vi "process_DAQ.vi"() -> ()   [LabVIEW 2011, in "Fiberscope_library.lvlib"]
uses:
  Fiberscope_library.lvlib
  typedefs/control_process_state_cluster.ctl
  typedefs/control_process_state_enum.ctl
  typedefs/fpga_main_spiral_fpga_ref.ctl
  typedefs/element_streams_cluster.ctl
  typedefs/feedback_to_watchdog.ctl
  typedefs/feedback_from_process_enum.ctl
  fpga/typedefs/pixel_to_host_enum.ctl
  typedefs/run_mode_enum.ctl
  typedefs/main_state_cluster.ctl
  typedefs/main_state_enum.ctl
  typedefs/all_scan_parameters_cluster.ctl
  typedefs/fiber_parameters_cluster.ctl
  fpga/typedefs/ramp_type_enum.ctl
  typedefs/spiral_parameters_cluster.ctl
  typedefs/run_parameters_cluster.ctl
  typedefs/acquisition_parameters_cluster.ctl
  typedefs/image_size_I32.ctl
  typedefs/smooth_coeffs_cluster.ctl
  typedefs/storage_parameters_cluster.ctl
  typedefs/mapping_corrections_cluster.ctl
  typedefs/pockels_corrections_cluster.ctl
  <vilib>/Utility/error.llb/Error Cluster From Error Code.vi
  <vilib>/rvi/errors/niLvFpgaAdjustHostInterfaceError.vi
  <vilib>/FPGAPlugInAG/PXI-7813R/niLvFpga_Reset_PXI-7813R.vi
  <vilib>/rvi/interface/nirviReadWriteControl/nirviReadWriteControl.xnode
  FPGA Bitfiles/FiberscopeRK1107_FPGATarget_fpgamainspiral_0DF2A7CB.lvbitx
  <vilib>/rvi/interface/nirviMethod/nirviMethod.xnode
  <vilib>/FPGAPlugInAG/PXI-7813R/niLvFpga_ConfigureFifo_PXI-7813R.vi
  <vilib>/rvi/errors/niLvFpgaMergeErrorWithErrorCode.vi
  NiFpgaLv.dll
panel:
  out "Forth or back?":bool
  out "Frame no":u32
  out "Elements remaining in FIFO":cluster{"Ch0":u32, "Ch1":u32}
  out "Pixels per frame":u32=1 min=1 max=90000 step=1
  out "error out":errorcluster
  in  "error in":errorcluster
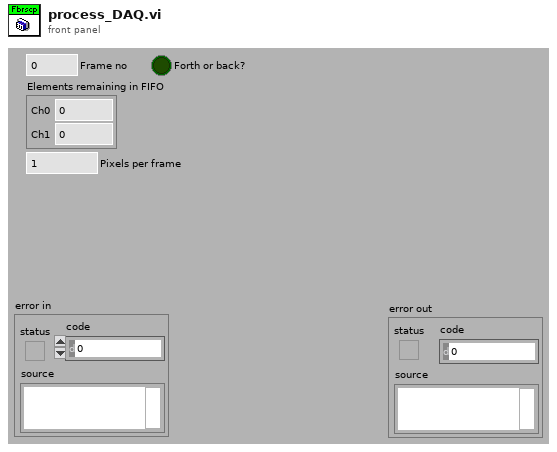
[diagram p1: front panel]
types:
  T1 = typedef "Fiberscope_library.lvlib/feedback_to_watchdog.ctl" = cluster{"Feedback_from_process_enum":T2, "Process_name":string}
  T2 = typedef "Fiberscope_library.lvlib/feedback_from_process_enum.ctl" = enum16{"Has_initialised", "Changed_parameters", "Has_started", "Has_stopped", "Has_quitted", "Is_running", "Has_finished", "Custom"}
  T3 = typedef "Fiberscope_library.lvlib/fpga_main_spiral_fpga_ref.ctl" = refnum<k20>
  T4 = typedef "Fiberscope_library.lvlib/control_process_state_cluster.ctl" = cluster{"Control_process_state_enum":T5, "variant":variant}
  T5 = typedef "Fiberscope_library.lvlib/control_process_state_enum.ctl" = enum16{"Init", "Quit", "Start", "Stop", "Change_parameters", "Running", "Finish", "Custom"}
  T6 = typedef "Fiberscope_library.lvlib/element_streams_cluster.ctl" = cluster{"Streams_array":dbl[][], "#channels":i32, "Last element?":bool, "Forth (1) or back (0)?":bool}
  T7 = typedef "pixel_to_host_enum.ctl" = enum16{"four-channel mode", "two-channel mode"}
  T8 = typedef "Fiberscope_library.lvlib/main_state_cluster.ctl" = cluster{"Main_state_enum":T9, "State_data_variant":variant}
  T9 = typedef "Fiberscope_library.lvlib/main_state_enum.ctl" = enum16{"Init", "Error", "Quit", "Run", "Stop", "Change_parameters", "Timeout", "Shutter", "Save", "Wait_for_finished", "Change_storage", "Change_pixelmap", "Change_averages", "Run_finished", "Change_runmode", "PMT"}
  T10 = typedef "Fiberscope_library.lvlib/run_mode_enum.ctl" = enum16{"Continuous", "Single frame", "No. of frames"}
  T11 = typedef "Fiberscope_library.lvlib/all_scan_parameters_cluster.ctl" = cluster{"Fiber parameters":T12, "Spiral parameters":T14, "Run parameters":T15, "Acquisition parameters":T16, "Fiber parameters pixel_mapper":T12, "Smooth_coeffs_cluster":T18, "Storage parameters":T19, "Mapping corrections":T20, "Pockels corrections":T21}
  T12 = typedef "Fiberscope_library.lvlib/fiber_parameters_cluster.ctl" = cluster{"Frequency":dbl, "Amplitude X":dbl, "Amplitude Y":dbl, "Initial Amplitude X":dbl, "Initial Amplitude Y":dbl, "Phase":dbl, "Ramp type":T13}
  T13 = typedef "ramp_type_enum.ctl" = enum8{"Linear", "Sine"}
  T14 = typedef "Fiberscope_library.lvlib/spiral_parameters_cluster.ctl" = cluster{"Imaging periods":dbl, "Settling periods":dbl, "Resting periods":dbl}
  T15 = typedef "Fiberscope_library.lvlib/run_parameters_cluster.ctl" = cluster{"Run mode":T10, "Averages per frame":u8, "No. of frames":u32}
  T16 = typedef "Fiberscope_library.lvlib/acquisition_parameters_cluster.ctl" = cluster{"Cycles per pixel":u32, "Image size":T17, "Bidirectional acquisition":bool}
  T17 = typedef "Fiberscope_library.lvlib/image_size_I32.ctl" = i32
  T18 = typedef "Fiberscope_library.lvlib/smooth_coeffs_cluster.ctl" = cluster{"Coeff 1":dbl, "Coeff 2":dbl}
  T19 = typedef "Fiberscope_library.lvlib/storage_parameters_cluster.ctl" = cluster{"Autosave":bool, "Path":path}
  T20 = typedef "Fiberscope_library.lvlib/mapping_corrections_cluster.ctl" = cluster{"Phase increase":dbl, "Amplitude correction":dbl}
  T21 = typedef "Fiberscope_library.lvlib/pockels_corrections_cluster.ctl" = cluster{"Delay pixels":i32}
  T22 = cluster{"Elements Remaining":u32, "Elements Remaining":u32}
  T23 = typedef "Fiberscope_library.lvlib/FPGA_acquisition_parameters.ctl" = cluster{"Cycles per pixel":u32, "Bitshift":i8, "Bidirectional acquisition":bool}
  T24 = typedef "scan_parameters_cluster.ctl" = cluster{"No. of waveforms":u16, "Continuous scanning":bool}
  T25 = typedef "cycle_parameters_XY_cluster.ctl" = cluster{"Cycle parameters X":T26, "Cycle parameters Y":T26}
  T26 = typedef "cycle_parameters_cluster.ctl" = cluster{"Imaging cycles":i32, "Settling cycles":i32, "Resting cycles":i32, "Phase advance per cycle":fxp<+,32,0>, "Initial Phase":fxp<+,32,1>}
  T27 = typedef "ramp_parameters_XY_cluster.ctl" = cluster{"Ramp parameters X":T28, "Ramp parameters Y":T28}
  T28 = typedef "ramp_parameters_cluster.ctl" = cluster{"Ramp type":T13, "Linear ramp parameters":T29, "Sine ramp parameters":T30}
  T29 = typedef "linear_ramp_parameters_cluster.ctl" = cluster{"Imaging multiplier advance per cycle":fxp<+/-,32,0>, "Settling multiplier advance per cycle":fxp<+/-,32,0>, "Imaging initial multiplier":fxp<+/-,43,12>}
  T30 = typedef "sine_ramp_parameters_cluster.ctl" = cluster{"Imaging phase advance per cycle":fxp<+,32,0>, "Settling phase advance per cycle":fxp<+,32,0>, "Scaler":fxp<+,43,12>, "Imaging initial phase":fxp<+,32,1>}
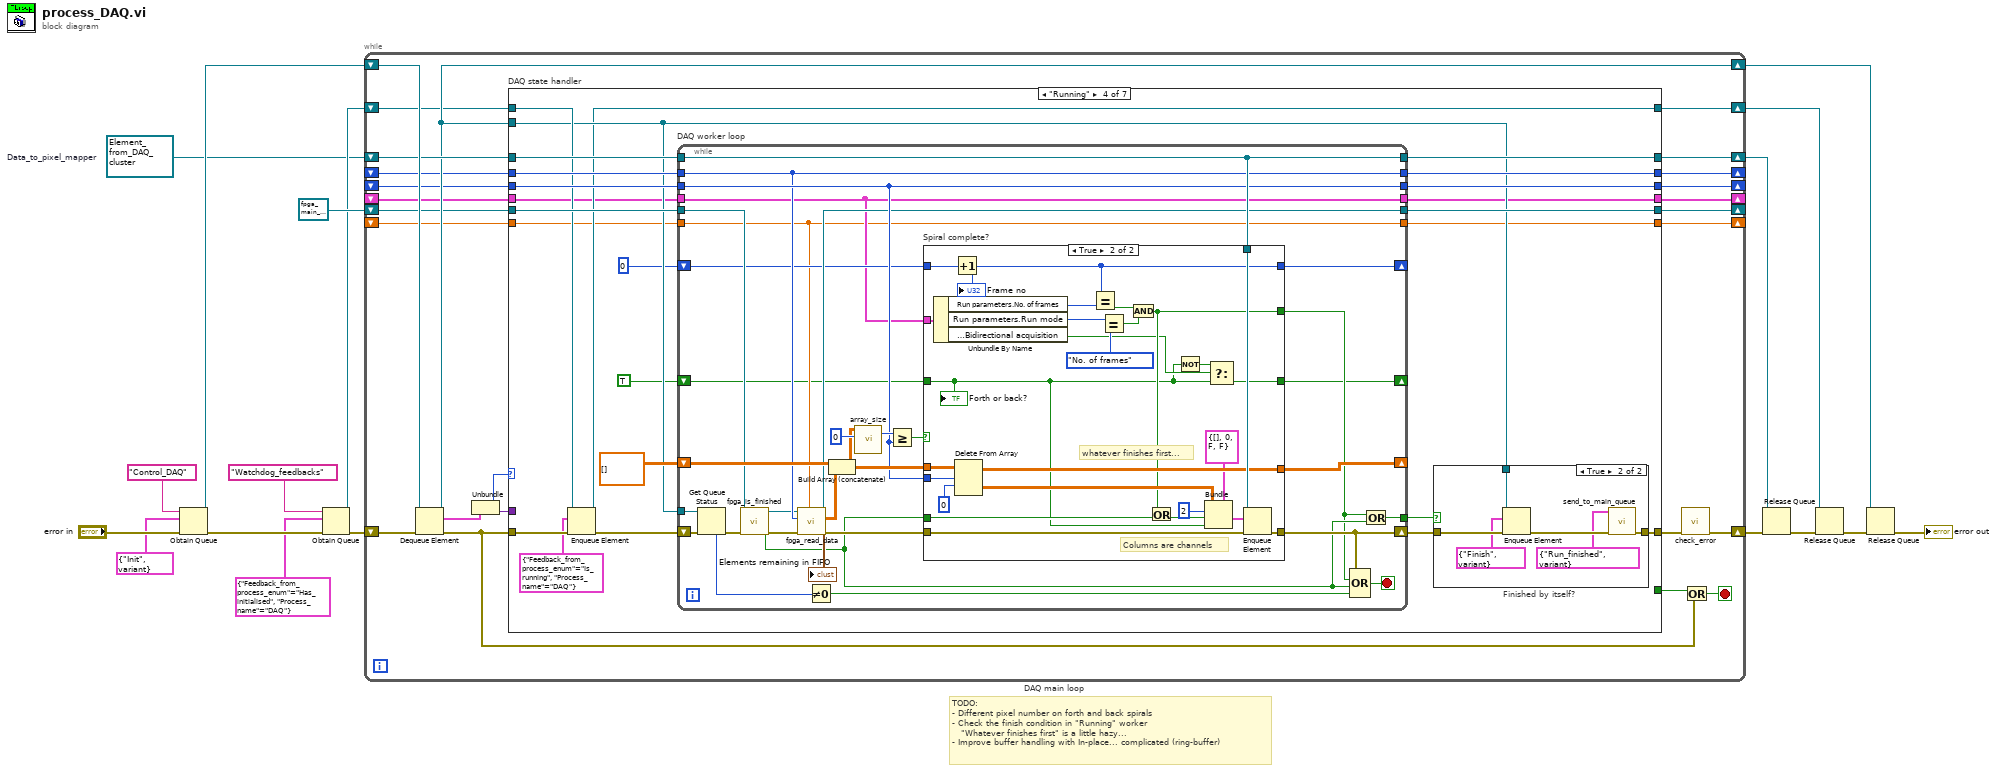
[diagram p0: block diagram]
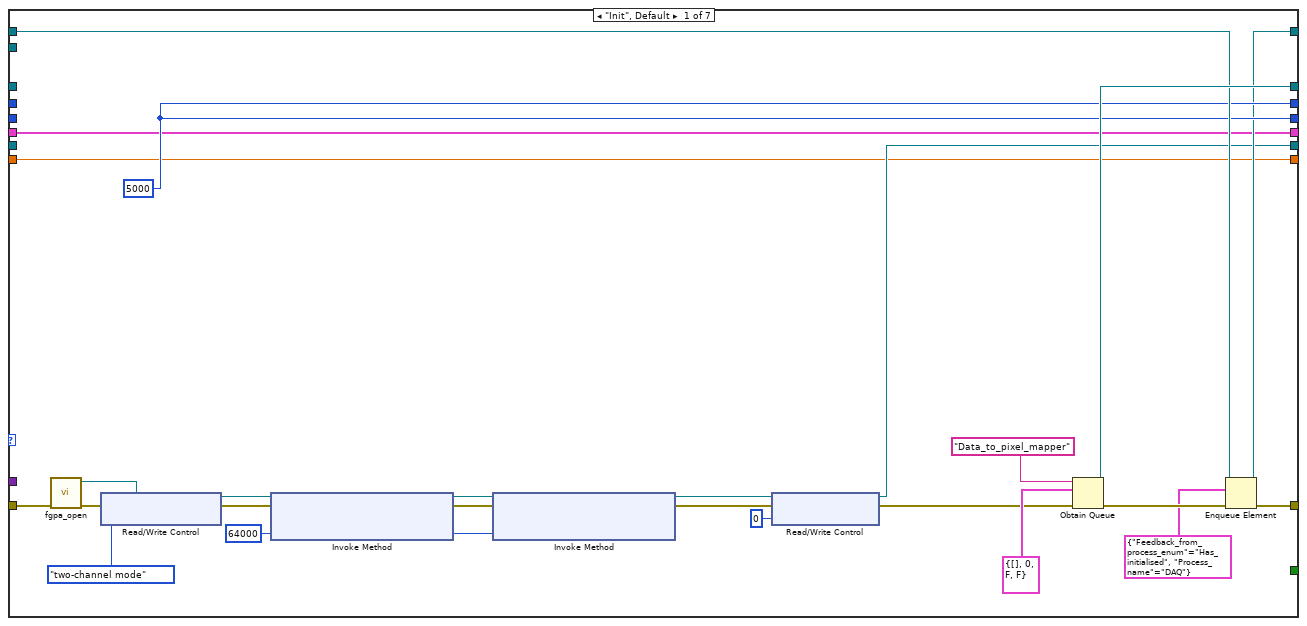
[diagram p2: hidden frame]
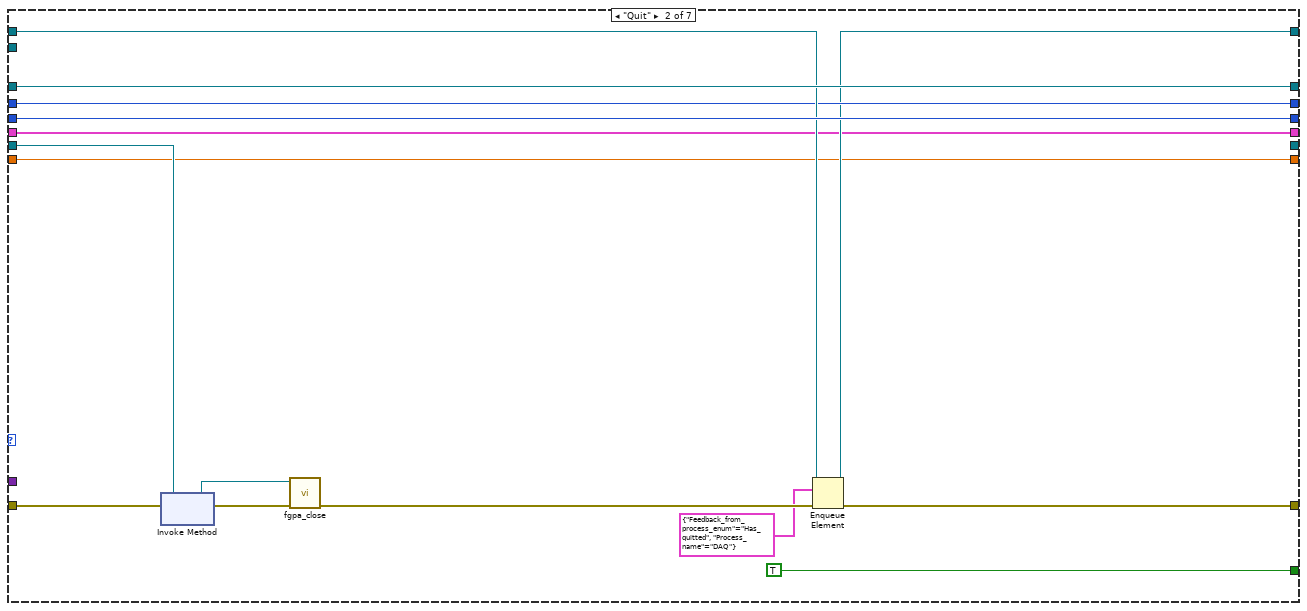
[diagram p3: hidden frame]
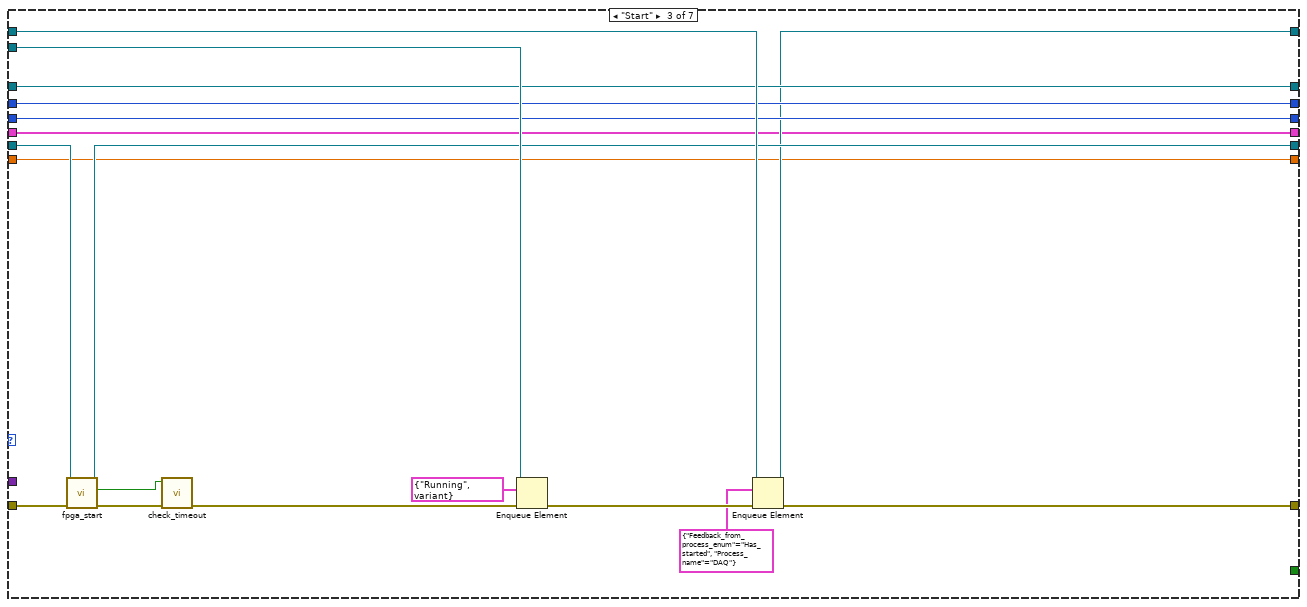
[diagram p4: hidden frame]
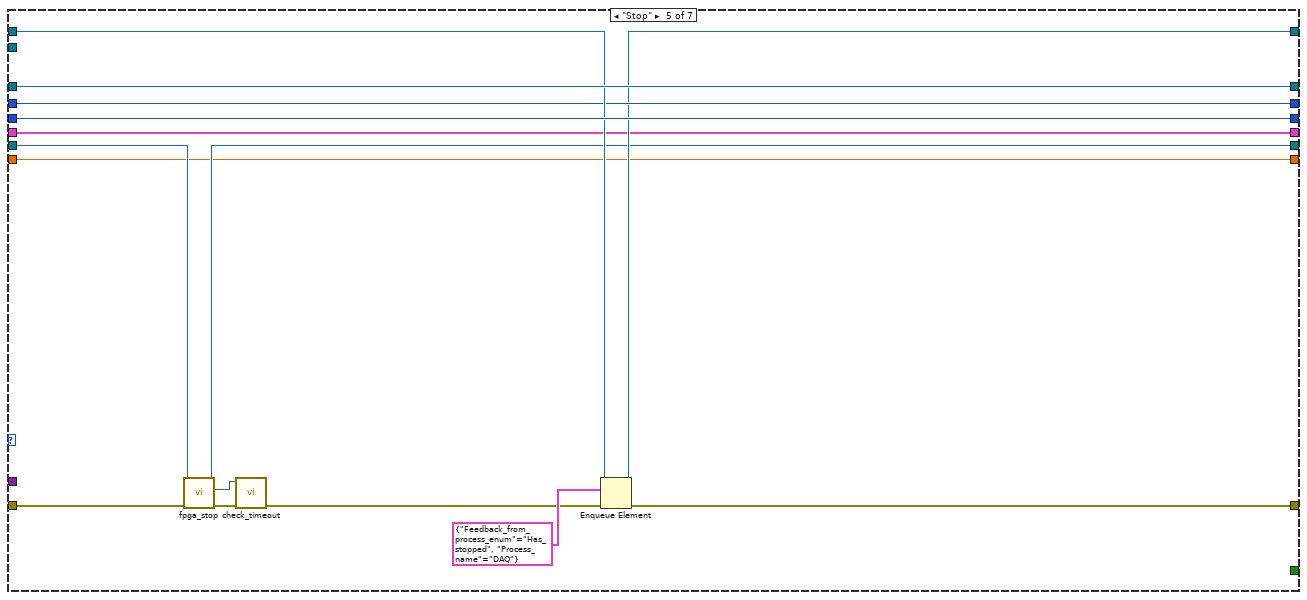
[diagram p7: hidden frame]
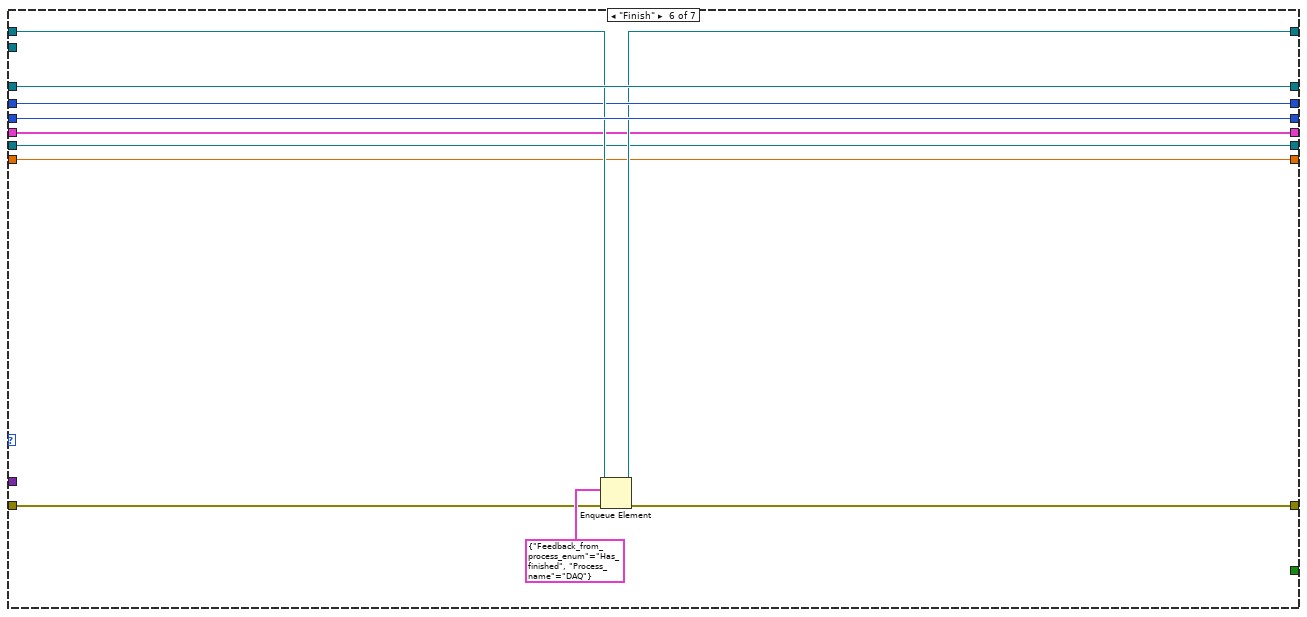
[diagram p8: hidden frame]
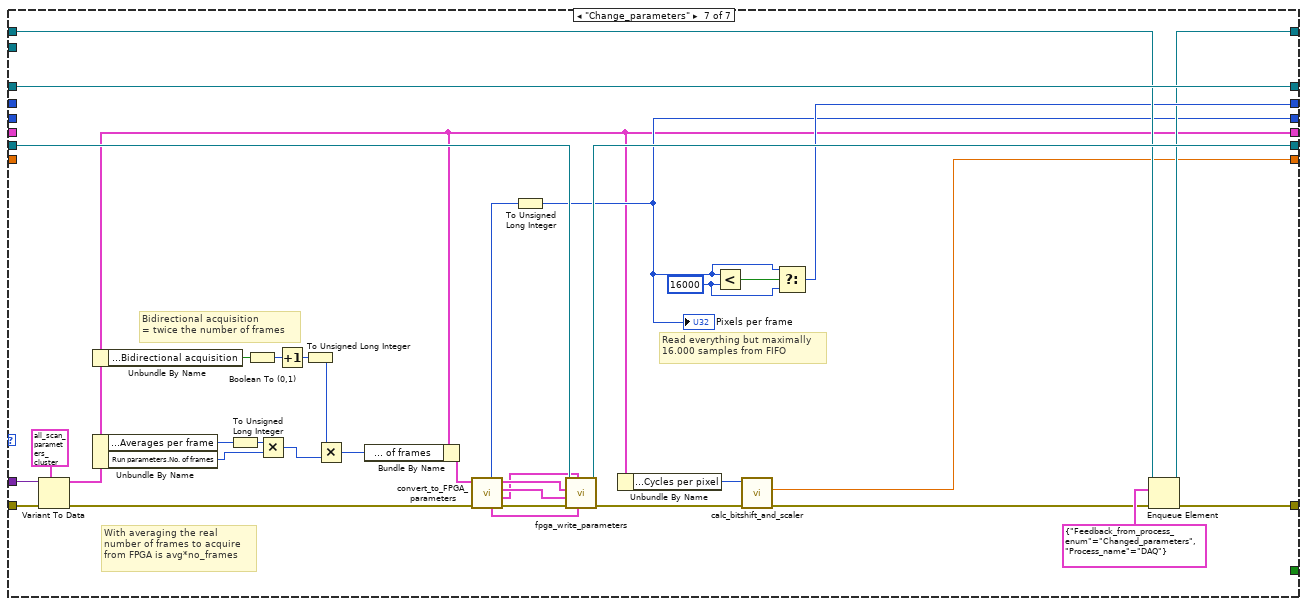
[diagram p9: hidden frame]
diagram:
  w2 = refnum<queue> refnum  # Data_to_pixel_mapper
  # "TODO:\n- Different pixel number on forth and back spirals \n- Check the finish condition in \"Running\" worker\n   \"Whatever finishes first\" is a little hazy...\n- Improve buffer handling with In-place... complicated (ring-buffer)"
  n1 = Obtain Queue(name (unnamed)="Control_DAQ", element data type=T4 {"Control_process_state_enum"=enum."Init", "variant"=variant} ("Control_process_state_cluster"), error in (no error)="error in") -> (queue out=w16:refnum<queue>, error out=w11:errorcluster)  [unwired: 2 in, 1 out]
  n2 = Obtain Queue(name (unnamed)="Watchdog_feedbacks", element data type=T1 {"Feedback_from_process_enum"=enum."Has_initialised", "Process_name"="DAQ"}, error in (no error)=w11) -> (queue out=w8:refnum<queue>, error out=w10:errorcluster)  [unwired: 2 in, 1 out]
  n3 = while "DAQ main loop" {
    shift-right: [w36] -> w5
    shift-left: w10 -> [w43]
    shift-right: [w33] -> w14
    shift-left: w16 -> [w42]
    shift-right: [w34] -> w3
    shift-left: w2 -> [w35]
    shift-right: [w32] -> _
    shift-left: T3 refnum ("FPGA VI Reference Out") -> [w31]
    shift-right: [w30] -> _
    shift-left: _ -> [w29]
    shift-right: [w23] -> w6
    shift-left: w8 -> [w28]
    shift-right: [w27] -> _
    shift-left: _ -> [w26]
    shift-right: [w22] -> _
    shift-left: _ -> [w21]
    shift-right: [w20] -> _
    shift-left: _ -> [w19]
    stop <- w39 stop-if-true
    n4 = Dequeue Element(queue=w42, error in (no error)=w43) -> (queue out=w33:refnum<queue>, element=w41:T4, error out=w24:errorcluster)  [unwired: 1 in, 1 out]
    n5 = Unbundle(w41) -> ("Control_process_state_enum"=w38:T5, "variant"=w40:variant)
    n6 = case "DAQ state handler" shown="\"Running\"" w38 {
      tunnel: w24 -> [w66 w80 w101 w116 w202 w211 w255]
      tunnel: [w63 w75 w96 w112 w207 w218 w246] -> w37
      tunnel: w40 -> [_ _ _ _ _ _ w254]
      tunnel: w35 -> [_ w83 w92 w121 w209 w220 w256]
      tunnel: [w67 w83 w92 w120 w209 w220 w256] -> w34
      tunnel: w33 -> [_ _ w94 w110 _ _ _]
      tunnel: [w45 _ w89 w117 w197 w212 w249] -> w32
      tunnel: w31 -> [_ w78 w100 w124 w201 w212 w250]
      tunnel: [w61 w82 w90 w118 w208 w219 w230] -> w30
      tunnel: w29 -> [_ w82 w90 w123 w208 w219 _]
      tunnel: [_ TRUE _ _ _ _ _] -> w25
      tunnel: w28 -> [w62 w74 w97 w114 w206 w217 w245]
      tunnel: [w61 w73 w91 w119 w205 w216 w242] -> w27
      tunnel: w26 -> [_ w73 w91 w122 w205 w216 _]
      tunnel: [w57 w72 w88 w109 w200 w215 w241] -> w23
      tunnel: [w50 w70 w86 w106 w198 w213 w229] -> w22
      tunnel: w21 -> [w50 w70 w86 w105 w198 w213 _]
      tunnel: [w44 w69 w84 w103 w195 w210 w232] -> w20
      tunnel: w19 -> [w44 w69 w84 w104 w195 w210 _]
      frame "Init", Default {
        w51 = u32 64000 ("Depth")
        w61 = 5000 ("Pixels per spiral")
        n7 = call "fgpa_open.vi"("error in"=w66) -> ("error out"=w60:errorcluster, "FPGA VI Reference Out"=w59:T3)  [unwired: 9 in]
        n8 = xnode "Read/Write Control"("FPGA VI Reference In"=w59, "error in"=w60, "pixel-to-host mode"=pixel_to_host_enum."two-channel mode") -> ("FPGA VI Reference Out"=w54:T3, "error out"=w55:errorcluster)
        n9 = xnode "Invoke Method"("FPGA VI Reference In"=w54, "error in"=w55, "Depth"=w51) -> ("FPGA VI Reference Out"=w52:T3, "error out"=w53:errorcluster)
        n10 = xnode "Invoke Method"("FPGA VI Reference In"=w52, "error in"=w53, "Depth"=w51) -> ("FPGA VI Reference Out"=w47:T3, "error out"=w49:errorcluster)
        n11 = xnode "Read/Write Control"("FPGA VI Reference In"=w47, "error in"=w49, "ADC clock phase"=u8 0) -> ("FPGA VI Reference Out"=w45:T3, "error out"=w48:errorcluster)
        n12 = Obtain Queue(name (unnamed)="Data_to_pixel_mapper", element data type=T6 {"Streams_array"=[], "#channels"=0, "Last element?"=FALSE, "Forth (1) or back (0)?"=FALSE} ("Element_from_DAQ_cluster"), error in (no error)=w48) -> (queue out=w67:refnum<queue>, error out=w64:errorcluster)  [unwired: 2 in, 1 out]
        n13 = Enqueue Element(queue=w62, element=T1 {"Feedback_from_process_enum"=enum."Has_initialised", "Process_name"="DAQ"}, error in (no error)=w64) -> (queue out=w57:refnum<queue>, error out=w63:errorcluster)  [unwired: 1 in, 1 out]
      }
      frame "Quit" {
        n14 = xnode "Invoke Method"("FPGA VI Reference In"=w78, "error in"=w80) -> ("FPGA VI Reference Out"=w77:T3, "error out"=w79:errorcluster)
        n15 = call "fgpa_close.vi"("error in"=w79, "FPGA VI Reference In"=w77) -> ("error out"=w76:errorcluster)  [unwired: 9 in]
        n16 = Enqueue Element(queue=w74, element=T1 {"Feedback_from_process_enum"=enum."Has_quitted", "Process_name"="DAQ"}, error in (no error)=w76) -> (queue out=w72:refnum<queue>, error out=w75:errorcluster)  [unwired: 1 in, 1 out]
      }
      frame "Start" {
        n17 = call "fpga_start.vi"("error in"=w101, "FPGA VI Reference in"=w100) -> ("error out"=w99:errorcluster, "Timed out?"=w98:bool, "FPGA VI Reference out"=w89:T3)  [unwired: 7 in]
        n18 = call "check_timeout.vi"("error in"=w99, "Timeout?"=w98) -> ("error out"=w85:errorcluster)  [unwired: 9 in]
        n19 = Enqueue Element(queue=w94, element=T4 {"Control_process_state_enum"=enum."Running", "variant"=variant}, error in (no error)=w85) -> (error out=w95:errorcluster)  [unwired: 1 in, 2 out]
        n20 = Enqueue Element(queue=w97, element=T1 {"Feedback_from_process_enum"=enum."Has_started", "Process_name"="DAQ"}, error in (no error)=w95) -> (queue out=w88:refnum<queue>, error out=w96:errorcluster)  [unwired: 1 in, 1 out]
      }
      frame "Running" {
        n21 = Enqueue Element(queue=w114, element=T1 {"Feedback_from_process_enum"=enum."Is_running", "Process_name"="DAQ"}, error in (no error)=w116) -> (queue out=w109:refnum<queue>, error out=w115:errorcluster)  [unwired: 1 in, 1 out]
        n22 = while "DAQ worker loop" {
          tunnel: w110 -> [w163]
          shift-right: [w139] -> w113
          shift-left: w115 -> [w164]
          tunnel: w124 -> [w147]
          tunnel: [w143] -> w117
          shift-right: [w156] -> _
          shift-left: dbl[][] [] ("Raw_streams_array") -> [w155]
          tunnel: [w159] -> w120
          tunnel: w121 -> [w159]
          tunnel: w123 -> [w151]
          tunnel: [w151] -> w118
          tunnel: [w150] -> w119
          tunnel: w122 -> [w150]
          tunnel: [w136] -> w111
          shift-right: [w141] -> _
          shift-left: u32 0 -> [w142]
          tunnel: w105 -> [w140]
          tunnel: [w140] -> w106
          tunnel: w104 -> [w135]
          tunnel: [w135] -> w103
          shift-right: [w133] -> _
          shift-left: TRUE -> [w134]
          stop <- w162 stop-if-true
          n23 = Get Queue Status(queue=w163, error in (no error)=w164) -> (error out=w148:errorcluster, # elements in queue=w153:i32)  [unwired: 1 in, 6 out]
          n24 = call "fpga_is_finished.vi"("error in"=w148, "FPGA VI Reference in"=w147) -> ("error out"=w146:errorcluster, "Finished?"=w138:bool, "FPGA VI Reference out"=w145:T3)  [unwired: 7 in]
          n25 = call "fpga_read_data.vi"("Scaler"=w135, "error in"=w146, "Number of Elements"=w150, "FPGA VI Reference in"=w145) -> ("error out"=w144:errorcluster, "Elements remaining"=→"Elements remaining in FIFO":T22, "Raw_streams_array"=w154:dbl[][], "FPGA VI Reference Out"=w143:T3)  [unwired: 4 in]
          n26 = Not Equal To 0?(x=w153) -> (x != 0?=w149:bool)
          n27 = Build Array (concatenate)(w155, w154) -> (w157:dbl[][])
          n28 = call "array_size.vi"("Array"=w157, "Dimension"=0) -> ("Dimension size"=w160:i32)  [unwired: 4 in]
          n29 = Greater Or Equal?(x=w160, y=w151) -> (x >= y?=w158:bool)
          n30 = case "Spiral complete?" shown="True" w158 {
            tunnel: [w167 w186] -> w139
            tunnel: w144 -> [w167 w194]
            tunnel: w159 -> [_ w193]
            tunnel: w157 -> [w168 w192]
            tunnel: [w168 w191] -> w156
            tunnel: w151 -> [_ w190]
            tunnel: w138 -> [_ w174]
            tunnel: w142 -> [w166 w183]
            tunnel: [w166 w182] -> w141
            tunnel: w140 -> [_ w181]
            tunnel: [_ w175] -> w137
            tunnel: w134 -> [w165 w169]
            tunnel: [w165 w171] -> w133
            frame False {
            }
            frame True {
              # "whatever finishes first..."
              # "Columns are channels"
              n31 = Unbundle By Name(w181) -> ("Run parameters.No. of frames"=w180:u32, "Run parameters.Run mode"=w179:T10, "Acquisition parameters.Bidirectional acquisition"=w172:bool)
              n32 = Increment(x=w183) -> (x+1=w182:u32)
              "Frame no" <- w182
              n33 = Delete From Array(array=w192, length=w190, index (row)=0) -> (deleted portion=w187:dbl[][], array with subset deleted=w191:dbl[][])  [unwired: 1 in]
              n34 = Equal?(x=w182, y=w180) -> (x = y?=w176:bool)
              n35 = Equal?(x=w179, y=run_mode_enum."No. of frames") -> (x = y?=w177:bool)
              n36 = And(x=w176, y=w177) -> (x .and. y?=w175:bool)
              n37 = Or(x=w175, y=w174) -> (x .or. y?=w173:bool)
              n38 = Not(x=w169) -> (.not. x?=w170:bool)
              n39 = Bundle(cluster=T6 {"Streams_array"=[], "#channels"=0, "Last element?"=FALSE, "Forth (1) or back (0)?"=FALSE} ("Element_from_DAQ_cluster"), "Streams_array"=w187, "#channels"=2, "Last element?"=w173, "Forth (1) or back (0)?"=w169) -> (w184:T6)
              n40 = Select(t=w170, s=w172, f=w169) -> (s? t:f=w171:bool)
              n41 = Enqueue Element(queue=w193, element=w184, error in (no error)=w194) -> (error out=w186:errorcluster)  [unwired: 1 in, 2 out]
              "Forth or back?" <- w169
            }
          }
          n42 = Compound Arithmetic op=OR(w139, w137, w138, w149) -> (w162:bool)
          n43 = Or(x=w137, y=w138) -> (x .or. y?=w136:bool)
        }
        n44 = case "Finished by itself?" shown="True" w111 {
          tunnel: w113 -> [w126 w132]
          tunnel: [w126 w128] -> w112
          tunnel: w110 -> [_ w131]
          frame False {
          }
          frame True {
            n45 = Enqueue Element(queue=w131, element=T4 {"Control_process_state_enum"=enum."Finish", "variant"=variant}, error in (no error)=w132) -> (error out=w129:errorcluster)  [unwired: 1 in, 2 out]
            n46 = call "send_to_main_queue.vi"("error in (no error)"=w129, "Main_state_cluster"=T8 {"Main_state_enum"=enum."Run_finished", "State_data_variant"=variant}) -> ("error out"=w128:errorcluster)  [unwired: 9 in]
          }
        }
      }
      frame "Stop" {
        n47 = call "fpga_stop.vi"("error in"=w202, "FPGA VI Reference in"=w201) -> ("error out"=w204:errorcluster, "Timed out?"=w203:bool, "FPGA VI Reference out"=w197:T3)  [unwired: 7 in]
        n48 = call "check_timeout.vi"("error in"=w204, "Timeout?"=w203) -> ("error out"=w196:errorcluster)  [unwired: 9 in]
        n49 = Enqueue Element(queue=w206, element=T1 {"Feedback_from_process_enum"=enum."Has_stopped", "Process_name"="DAQ"}, error in (no error)=w196) -> (queue out=w200:refnum<queue>, error out=w207:errorcluster)  [unwired: 1 in, 1 out]
      }
      frame "Finish" {
        n50 = Enqueue Element(queue=w217, element=T1 {"Feedback_from_process_enum"=enum."Has_finished", "Process_name"="DAQ"}, error in (no error)=w211) -> (queue out=w215:refnum<queue>, error out=w218:errorcluster)  [unwired: 1 in, 1 out]
      }
      frame "Change_parameters" {
        w243 = u32 16000 ("y")
        # "Read everything but maximally\n16.000 samples from FIFO"
        # "Bidirectional acquisition\n= twice the number of frames"
        # "With averaging the real\nnumber of frames to acquire\nfrom FPGA is avg*no_frames"
        n51 = Variant To Data(error in=w255, type=T11 {"Fiber parameters"={"Frequency"=100.0, "Amplitude X"=0.0, "Amplitude Y"=0.0, "Initial Amplitude X"=0.0, "Initial Amplitude Y"=0.0, "Phase"=0.0, "Ramp type"=enum."Linear"}, "Spiral parameters"={"Imaging periods"=1.0, "Settling periods"=1.0, "Resting periods"=1.0}, "Run parameters"={"Run mode"=enum."Continuous", "Averages per frame"=0, "No. of frames"=0}, "Acquisition parameters"={"Cycles per pixel"=0, "Image size"=1, "Bidirectional acquisition"=FALSE}, "Fiber parameters pixel_mapper"={"Frequency"=0.0, "Amplitude X"=0.0, "Amplitude Y"=0.0, "Initial Amplitude X"=0.0, "Initial Amplitude Y"=0.0, "Phase"=0.0, "Ramp type"=enum."Linear"}, "Smooth_coeffs_cluster"={"Coeff 1"=0.0, "Coeff 2"=0.0}, "Storage parameters"={"Autosave"=FALSE, "Path"=path ""}, "Mapping corrections"={"Phase increase"=0.0, "Amplitude correction"=0.0}, "Pockels corrections"={"Delay pixels"=0}} ("All scan parameters"), Variant=w254) -> (data=w229:T11, error out=w252:errorcluster)
        n52 = Unbundle By Name(w229) -> ("Acquisition parameters.Bidirectional acquisition"=w228:bool)
        n53 = Unbundle By Name(w229) -> ("Run parameters.Averages per frame"=w237:u8, "Run parameters.No. of frames"=w238:u32)
        n54 = To Unsigned Long Integer(number=w237) -> (unsigned 32bit integer=w236:u32)
        n55 = Boolean To (0,1)(Boolean=w228) -> (0, 1=w227:i16)
        n56 = Multiply(x=w236, y=w238) -> (x*y=w226:u32)
        n57 = Increment(x=w227) -> (x+1=w224:i16)
        n58 = To Unsigned Long Integer(number=w224) -> (unsigned 32bit integer=w223:u32)
        n59 = Multiply(x=w223, y=w226) -> (x*y=w225:u32)
        n60 = Bundle By Name(cluster=w229, "Run parameters.No. of frames"=w225) -> (w239:T11)
        n61 = call "convert_to_FPGA_parameters.vi"("error in"=w252, "All scan parameters"=w239) -> ("error out"=w251:errorcluster, "FPGA_acquisition_parameters"=w222:T23, "FPGA Scan Parameters"=w247:T24, "FPGA cycle parameters XY"=w248:T25, "FPGA ramp parameters XY"=w221:T27, "Pixels per spiral"=w231:i32)  [unwired: 4 in]
        n62 = To Unsigned Long Integer(number=w231) -> (unsigned 32bit integer=w230:u32)
        "Pixels per frame" <- w230
        n63 = call "fpga_write_parameters.vi"("Ramp parameters XY"=w221, "FPGA_acquisition_parameters"=w222, "error in"=w251, "FPGA Scan Parameters"=w247, "FPGA Cycle Parameters XY"=w248, "FPGA VI Reference in"=w250) -> ("error out"=w234:errorcluster, "FPGA VI Reference Out"=w249:T3)  [unwired: 4 in]
        n64 = Unbundle By Name(w229) -> ("Acquisition parameters.Cycles per pixel"=w235:u32)
        n65 = Less?(x=w230, y=w243) -> (x < y?=w244:bool)
        n66 = call "calc_bitshift_and_scaler.vi"("error in"=w234, "Cycles per pixel"=w235) -> ("error out"=w233:errorcluster, "Scaler"=w232:dbl)  [unwired: 7 in, 1 out]
        n67 = Select(t=w230, s=w244, f=w243) -> (s? t:f=w242:u32)
        n68 = Enqueue Element(queue=w245, element=T1 {"Feedback_from_process_enum"=enum."Changed_parameters", "Process_name"="DAQ"}, error in (no error)=w233) -> (queue out=w241:refnum<queue>, error out=w246:errorcluster)  [unwired: 1 in, 1 out]
      }
    }
    n69 = call "check_error.vi"("error in"=w37) -> ("error out"=w36:errorcluster)  [unwired: 10 in]
    n70 = Or(x=w25, y=w24) -> (x .or. y?=w39:bool)
  }
  n71 = Release Queue(queue=w3, error in (no error)=w5) -> (error out=w4:errorcluster)  [unwired: 1 in, 2 out]
  n72 = Release Queue(queue=w6, error in (no error)=w4) -> (error out=w7:errorcluster)  [unwired: 1 in, 2 out]
  n73 = Release Queue(queue=w14, error in (no error)=w7) -> (error out=→"error out":errorcluster)  [unwired: 1 in, 2 out]
